vi "brokenvi.vi"() -> ()   [LabVIEW 2021]
panel:
  out "x = y?":bool
  in  "y":dbl
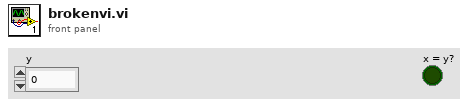
[diagram p1: front panel]
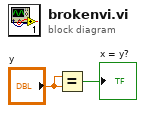
[diagram p0: block diagram]
diagram:
  n1 = Equal?(x="y", y="y") -> (x = y?=→"x = y?":bool)
